vi "3.1.15-Arbitrator Multiply.vi"(4 "Speed By Path 5":dbl[](array[numeric]), 5 "Speed By Path":sgl[](array[numeric]), 6 "Speed By Path 2":sgl[](array[numeric]), 7 "Speed By Path 3":sgl[](array[numeric]), 8 "Speed By Path 4":dbl[](array[numeric])) -> (0 "Index":i32, 1 "Max Speed":dbl, 3 "Arbitrated Output":dbl[](array[numeric]))   [LabVIEW 2010]
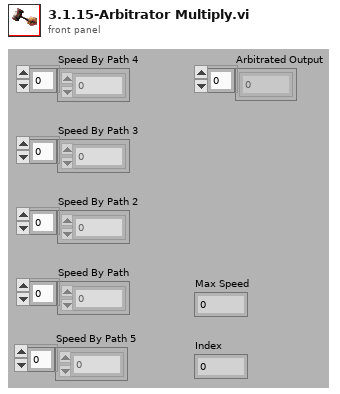
[diagram p1: front panel]
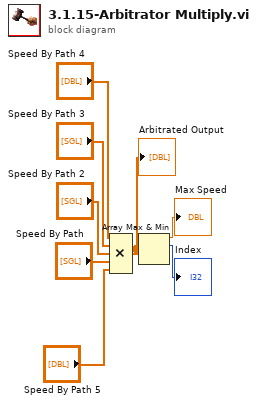
[diagram p0: block diagram]
diagram:
  n1 = Compound Arithmetic op=MULTIPLY("Speed By Path 4", "Speed By Path 3", "Speed By Path 2", "Speed By Path", "Speed By Path 5") -> (w8:dbl[])
  "Arbitrated Output" <- w8
  n2 = Array Max & Min(array=w8) -> (max value=→"Max Speed":dbl, max index (indices)=→"Index":i32)  [unwired: 2 out]
